vi "StringToComplexNumber.vi"(8 "error in (no error)":errorcluster, 11 "input string":string) -> (0 "error out":errorcluster, 3 "x + iy":cxt)   [LabVIEW 2021]
uses:
  <vilib>/regexp/Match Regular Expression.xnode
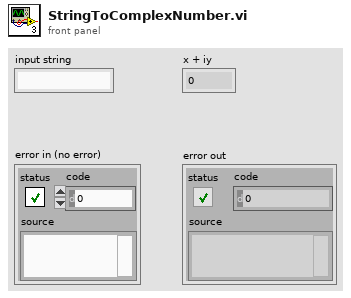
[diagram p1: front panel]
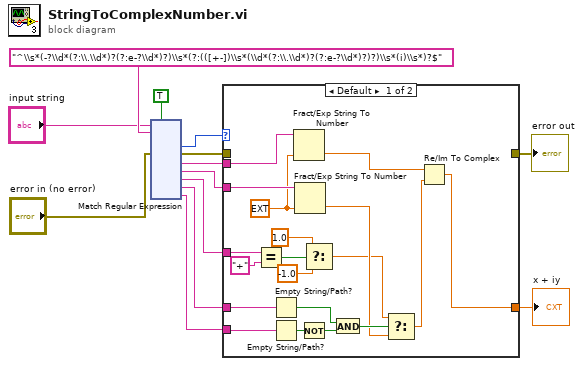
[diagram p0: block diagram]
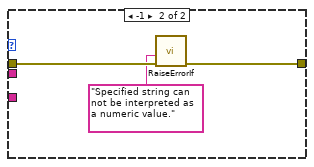
[diagram p2: hidden frame]
diagram:
  n1 = xnode "Match Regular Expression"("input string"="input string", "regular expression"="^\\s*(-?\\d*(?:\\.\\d*)?(?:e-?\\d*)?)\\s*(?:(([+-])\\s*(\\d*(?:\\.\\d*)?(?:e-?\\d*)?)?)\\s*(i)\\s*)?$", "error in"="error in (no error)", "ignore case? (F)"=TRUE) -> ("offset past match"=w11:i32, "error out"=w9:errorcluster, "submatch 1"=w6:string, "submatch 2"=w7:string, "submatch 3"=w1:string, "submatch 4"=w3:string, "submatch 5"=w2:string)  [unwired: 2 in, 3 out]
  n2 = case shown="Default" w11 {
    tunnel: w9 -> [_ w35]
    tunnel: [_ w33] -> w8
    tunnel: w7 -> [w28 _]
    tunnel: w6 -> [w32 _]
    tunnel: [w30 _] -> w5
    tunnel: w2 -> [w29 _]
    tunnel: w3 -> [w21 _]
    tunnel: w1 -> [w19 _]
    frame Default {
      w20 = ext 0.0 ("default (0 DBL)")
      n3 = Equal?(x=w19, y="+") -> (x = y?=w17:bool)
      n4 = Empty String/Path?(string/path=w21) -> (empty?=w25:bool)
      n5 = Empty String/Path?(string/path=w29) -> (empty?=w27:bool)
      n6 = Fract/Exp String To Number(string=w32, default (0 dbl)=w20) -> (number=w31:ext)  [unwired: 2 in, 1 out]
      n7 = Fract/Exp String To Number(string=w28, default (0 dbl)=w20) -> (number=w23:ext)  [unwired: 2 in, 1 out]
      n8 = Not(x=w27) -> (.not. x?=w26:bool)
      n9 = Select(t=1.0, s=w17, f=-1.0) -> (s? t:f=w14:dbl)
      n10 = And(x=w25, y=w26) -> (x .and. y?=w24:bool)
      n11 = Select(t=w14, s=w24, f=w23) -> (s? t:f=w22:ext)
      n12 = Re/Im To Complex(1:w22, 2:w31) -> (0:w30:cxt)
    }
    frame -1 {
      n13 = call "RaiseErrorIf.vi"("error in (no error)"=w35, "error message"="Specified string can not be interpreted as a numeric value.") -> ("error out"=w33:errorcluster)  [unwired: 9 in]
    }
  }
  "error out" <- w8
  "x + iy" <- w5
